vi "Parse.vi"(8 "Error In":errorcluster, 11 "object in":refnum<class "2021_16.lvclass">) -> (0 "Error Out":errorcluster, 3 "object out":refnum<class "2021_16.lvclass">)   [LabVIEW 2023, in "2021_16.lvclass"]
uses:
  2021_16.lvclass
  2021_16.lvclass/2021_16.ctl
  <vilib>/Utility/error.llb/Trim Whitespace One-Sided.vi
  <userlib>/_OpenG.lib/string/string.llb/openg_string.lvlib
panel:
  out "Data":bool[](array[boolean])
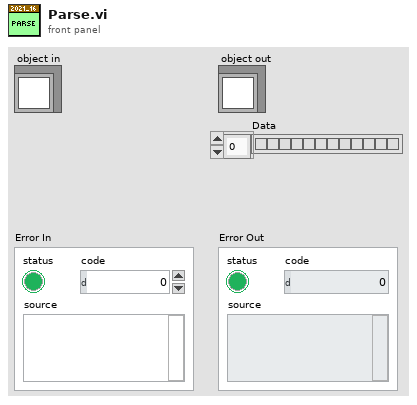
[diagram p1: front panel]
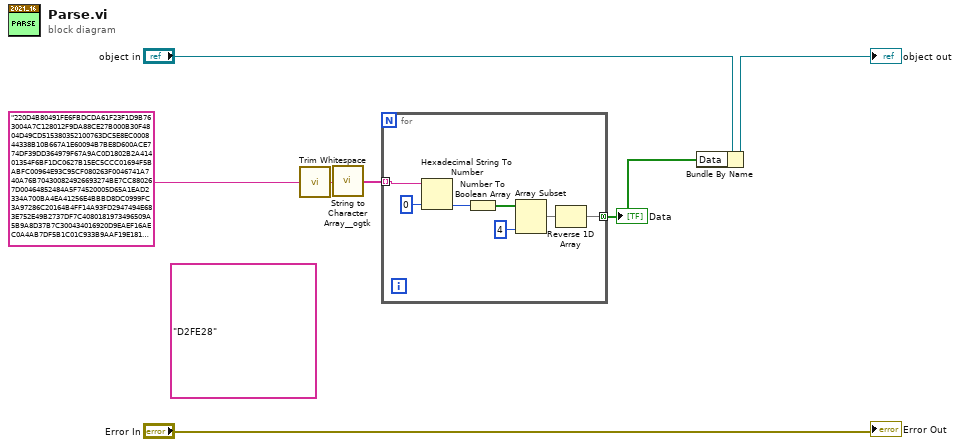
[diagram p0: block diagram]
diagram:
  (unwired) "D2FE28"
  n1 = call <vilib>:"Trim Whitespace.vi"("string"="220D4B80491FE6FBDCDA61F23F1D9B763004A7C128012F9DA88CE27B000B30F4804D49CD515380352100763DC5E8EC000844338B10B667A1E60094B7BE8D600ACE774DF39DD364979F67A9AC0D1802B2A41401354F6BF1DC0627B15EC5CCC01694F5BABFC00964E93C95CF080263F0046741A740A76B704300824926693274BE7CC880267D00464852484A5F74520005D65A1EAD2334A700BA4EA41256E4BBBD8DC0999FC3A97286C20164B4FF14A93FD2947494E683E752E49B2737DF7C4080181973496509A5B9A8D37B7C300434016920D9EAEF16AEC0A4AB7DF5B1C01C933B9AAF19E1818027A00A80021F1FA0E43400043E174638572B984B066401D3E802735A4A9ECE371789685AB3E0E800725333EFFBB4B8D131A9F39ED413A1720058F339EE32052D48EC4E5EC3...") -> ("trimmed string"=w4:string)  [unwired: 1 in]
  n2 = call <userlib>:"String to Character Array__ogtk.vi"("Input String"=w4) -> ("Character Array"=w3:string[])
  n3 = for {
    tunnel: w3 -> [w14] mode=indexing
    tunnel: [w8] -> w2 mode=concatenating
    n4 = Hexadecimal String To Number(string=w14, default (0uL)=u8 0 ("default (0 U32)")) -> (number=w12:u8)  [unwired: 1 in, 1 out]
    n5 = Number To Boolean Array(number=w12) -> (Boolean array=w11:bool[])
    n6 = Array Subset(array=w11, length=4) -> (w9:bool[])  [unwired: 1 in]
    n7 = Reverse 1D Array(array=w9) -> (reversed array=w8:bool[])
  }
  "Data" <- w2
  n8 = Bundle By Name(cluster="object in", "Data"=w2) -> (→"object out":refnum<class "2021_16.lvclass">)
  "Error Out" <- "Error In"
